vi "m1m3_getNextSample_GyroData.vi"(8 "error in (no error)":errorcluster, 11 "GyroData_Ctl":T1) -> (0 "error out":errorcluster, 2 "function return":i32, 3 "GyroData_Ctl out":T1)   [LabVIEW 2016, in "SALLV_m1m3.lvlib"]
doc: "int m1m3_shm_getNextSample_GyroDataLV(m1m3_GyroDataLV *GyroData_Ctl );"
uses:
  SALLV_m1m3.lvlib
  DataTypes/GyroData.ctl
  SALLV_m1m3.so
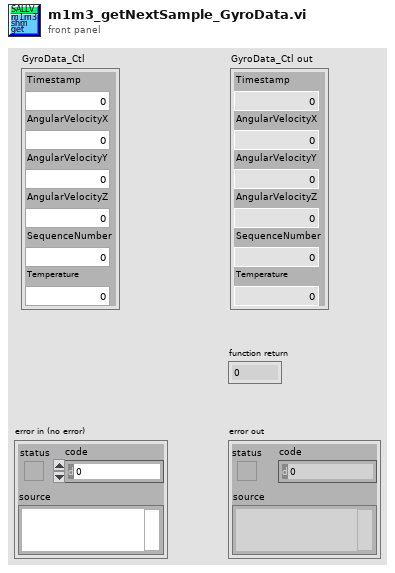
[diagram p1: front panel]
types:
  T1 = typedef "SALLV_m1m3.lvlib/GyroData.ctl" = cluster{"Timestamp":dbl, "AngularVelocityX":dbl, "AngularVelocityY":dbl, "AngularVelocityZ":dbl, "SequenceNumber":u8, "Temperature":i16}
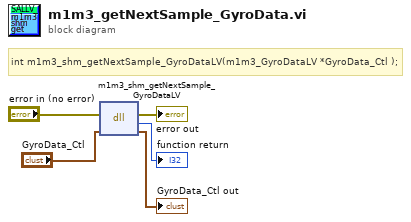
[diagram p0: block diagram]
diagram:
  # "int m1m3_shm_getNextSample_GyroDataLV(m1m3_GyroDataLV *GyroData_Ctl );"
  n1 = dll-call lib="opt/CODE/SALLV_m1m3/SALLV_m1m3.*" fn="m1m3_shm_getNextSample_GyroDataLV"(error in="error in (no error)", "GyroData_Ctl"="GyroData_Ctl") -> (error out=→"error out":errorcluster, →"function return":i32, "GyroData_Ctl"=→"GyroData_Ctl out":T1)  [unwired: 2 in, 1 out]
